vi "Testing.vi"() -> ()   [LabVIEW 2017, in "HMILibrary.lvlib"]
uses:
  HMILibrary.lvlib
panel:
  in  "stop":bool
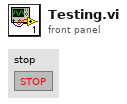
[diagram p1: front panel]
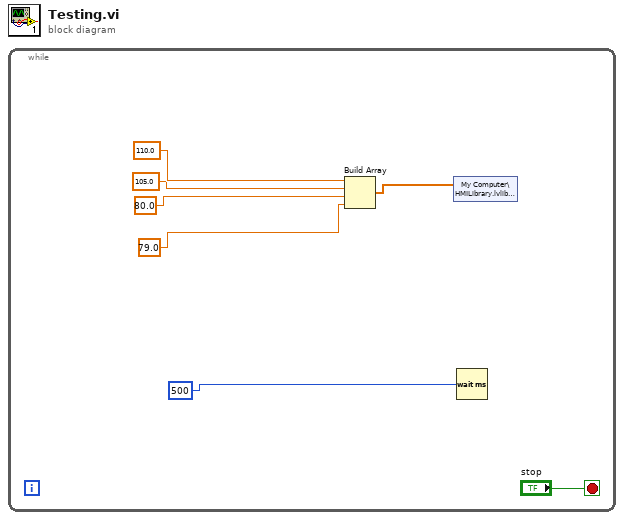
[diagram p0: block diagram]
diagram:
  n1 = while {
    stop <- "stop" stop-if-true
    n2 = Build Array(110.0, 105.0, 80.0, 79.0) -> (w2:dbl[])
    n3 = shared-variable "My Computer\\HMILibrary.lvlib\\T_n"(w2) -> ()  [unwired: 1 in, 1 out]
    n4 = Wait (ms)(milliseconds to wait=500) -> ()  [unwired: 1 out]
  }
